vi "Check Action.vi"(6 "HRS Time":dbl, 7 "Values In":dbl[](array[numeric]), 8 "error in (no error)":errorcluster, 11 "PulsedValve in":refnum<class "PulsedValve.lvclass">) -> (0 "error out":errorcluster, 1 "Do Action":bool, 2 "Action":T1, 3 "PulsedValve out":refnum<class "PulsedValve.lvclass">, 5 "Values":dbl[](array[numeric]))   [LabVIEW 2020, in "VolatusControl.lvlib" / "PulsedValve.lvclass"]
uses:
  PulsedValve.lvclass
  Valve Action.ctl
  Volatus/MessageQ/MessageQ.lvclass
  PulsedValve.lvclass/PulsedValve.ctl
  State.ctl
  VolatusControl.lvlib
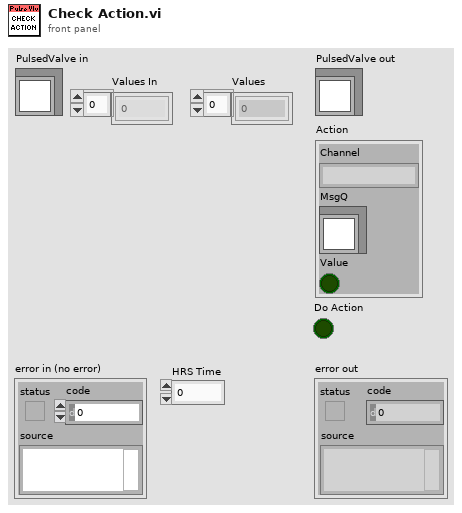
[diagram p1: front panel]
types:
  T1 = typedef "VolatusControl.lvlib/Valve Action.ctl" = cluster{"Channel":string, "MsgQ":refnum<class "MessageQ.lvclass">, "Value":bool}
  T2 = typedef "VolatusControl.lvlib/PulsedValve.lvclass/State.ctl" = enum16{"Idle", "Start", "On", "Off"}
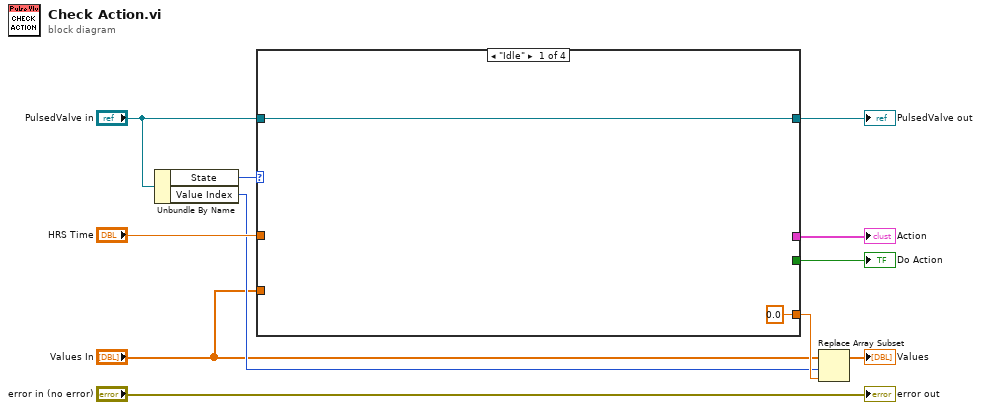
[diagram p0: block diagram]
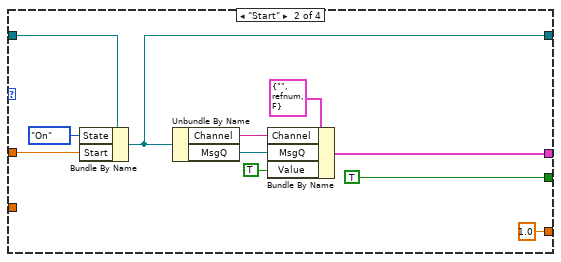
[diagram p2: hidden frame]
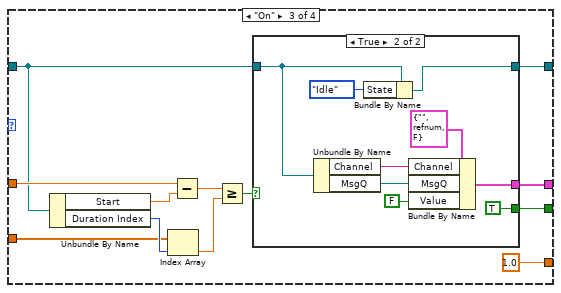
[diagram p3: hidden frame]
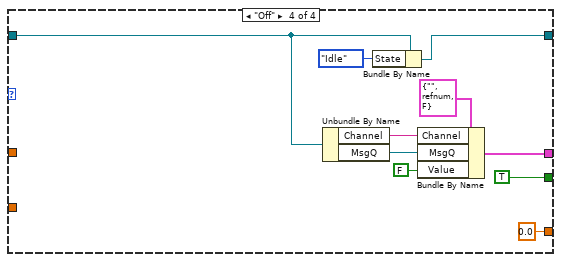
[diagram p5: hidden frame]
diagram:
  n1 = Unbundle By Name("PulsedValve in") -> ("State"=w10:T2, "Value Index"=w2:i32)
  n2 = case shown="\"Idle\"" w10 {
    tunnel: "HRS Time" -> [_ w24 w36 _]
    tunnel: "PulsedValve in" -> [w13 w22 w30 w51]
    tunnel: [w13 w20 w29 w50] -> w7
    tunnel: [_ w19 w33 w49] -> w6
    tunnel: [_ TRUE w32 TRUE] -> w5
    tunnel: [0.0 1.0 1.0 0.0] -> w3
    tunnel: "Values In" -> [_ _ w26 _]
    frame "Idle" {
    }
    frame "Start" {
      n3 = Bundle By Name(cluster=w22, "State"=State."On", "Start"=w24) -> (w20:refnum<class "PulsedValve.lvclass">)
      n4 = Unbundle By Name(w20) -> ("Channel"=w18:string, "MsgQ"=w17:refnum<class "MessageQ.lvclass">)
      n5 = Bundle By Name(cluster=T1 {"Channel"="", "MsgQ"=refnum, "Value"=FALSE} ("Action"), "Channel"=w18, "MsgQ"=w17, "Value"=TRUE) -> (w19:T1)
    }
    frame "On" {
      n6 = Unbundle By Name(w30) -> ("Start"=w35:dbl, "Duration Index"=w27:i32)
      n7 = Index Array(array=w26, index=w27) -> (element=w25:dbl)
      n8 = Subtract(x=w36, y=w35) -> (x-y=w34:dbl)
      n9 = Greater Or Equal?(x=w34, y=w25) -> (x >= y?=w31:bool)
      n10 = case shown="True" w31 {
        tunnel: [_ w42] -> w33
        tunnel: [_ TRUE] -> w32
        tunnel: w30 -> [w37 w40]
        tunnel: [w37 w38] -> w29
        frame False {
        }
        frame True {
          n11 = Unbundle By Name(w40) -> ("Channel"=w45:string, "MsgQ"=w44:refnum<class "MessageQ.lvclass">)
          n12 = Bundle By Name(cluster=w40, "State"=State."Idle") -> (w38:refnum<class "PulsedValve.lvclass">)
          n13 = Bundle By Name(cluster=T1 {"Channel"="", "MsgQ"=refnum, "Value"=FALSE} ("Action"), "Channel"=w45, "MsgQ"=w44, "Value"=FALSE) -> (w42:T1)
        }
      }
    }
    frame "Off" {
      n14 = Unbundle By Name(w51) -> ("Channel"=w55:string, "MsgQ"=w54:refnum<class "MessageQ.lvclass">)
      n15 = Bundle By Name(cluster=w51, "State"=State."Idle") -> (w50:refnum<class "PulsedValve.lvclass">)
      n16 = Bundle By Name(cluster=T1 {"Channel"="", "MsgQ"=refnum, "Value"=FALSE} ("Action"), "Channel"=w55, "MsgQ"=w54, "Value"=FALSE) -> (w49:T1)
    }
  }
  "PulsedValve out" <- w7
  "Action" <- w6
  "Do Action" <- w5
  n17 = Replace Array Subset(array="Values In", new element=w3, index=w2) -> (→"Values":dbl[])
  "error out" <- "error in (no error)"
